vi "8-Tap 8-bit Camera with Serial Server(FPGA).vi"() -> ()   [LabVIEW 2013]
doc: "This is the FPGA VI for the 10-Tap 8-Bit Camera with DRAM example. This example demonstrates how to acquire images from a 10-tap, 8-bit, extended configuration, Camera Link camera and transfer the images to the host. This example supports area scan and line scan cameras for both continuous and finite acquisitions.\n\nThis example also demonstrates the use of DRAM as a frame buffer for very high speed acquisitions. Data packing and flow-control are also employed to maximize use of the available DRAM and FIFOs in terms of both memory space and performance.\n\nAdditionally, the example demonstrates the serial server, which allows third-party camera configuration utilities to communicate with the camera using the Camera Link serial interface while this VI is running."
uses:
  Common/CL Signal Mapping.ctl
  Common/CL Configuration.ctl
  FPGA/Sector/Accumulate/Sector Parameter Cluster.ctl
  <vilib>/Platform/TimedLoop/XDataNode/timing_clust.ctl
  <vilib>/Platform/TimedLoop/XDataNode/nitl_modes.ctl
  <vilib>/Platform/TimedLoop/XDataNode/wakeup.ctl
  <vilib>/rvi/Emulation/niFpgaSctlEmulationGetInTimedLoop.vi
  <vilib>/rvi/Emulation/niFpgaEmulationReportErrorSimple.vi
  <vilib>/rvi/eio/common/nirviEmuTemplateMethod_errors.vi
  <vilib>/rvi/Emulation/niFpgaGetClockAttributes.vi
  <vilib>/rvi/Emulation/niFpgaCriticalErrorInLSC.vi
  Common/CL Data to Pixels/8 Tap 8-Bit.vi
  FPGA/Globals/Accumulated Sector Intensity.vi
  <vilib>/rvi/FIFO/Fifo_Resource/nirvififoEmulationWriteFpgaImpl.vi
  <vilib>/rvi/DataTransferAndStorage/Container/Common/niFpgaContainerGetUniqueNameForEmu.vi
  <vilib>/rvi/interface/RandomDataEmulation/nirviRandomDataFPGAFIFO.vi
  <vilib>/rvi/interface/RandomDataEmulation/niFpgaRandomDataHandleErrors.vi
  <vilib>/rvi/FIFO/Fifo_Resource/nirvififoEmulationGetNumberOfElementsToReadFpgaImpl.vi
  <vilib>/rvi/FIFO/Fifo_Resource/nirvififoEmulationGetNumberOfElementsToWriteFpgaImpl.vi
  <vilib>/rvi/FIFO/Fifo_Resource/nirvififoEmulationReadFpgaImpl.vi
  FPGA/Globals/Sector Parameter Global.vi
  <vilib>/rvi/Emulation/niFpgaProcessEmulError.vi
  FPGA/Globals/Pixel Location Global.vi
  <vilib>/Platform/TimedLoop/XDataNode/XDataNode.xnode
  <vilib>/eio/EIONode/EIONode.xnode
  <vilib>/rvi/DataTransferAndStorage/Container/XNode/niFpgaContainer.xnode
  <vilib>/rvi/FIFO/Fifo_Resource/nirvififoEmulationWrite.vi
  <vilib>/rvi/interface/RandomDataEmulation/nirviRandomDataFpgaReadWriteTemplate.vi
  <vilib>/rvi/FIFO/Fifo_Resource/nirvififoEmulationGetNumberOfElementsToRead.vi
  <vilib>/rvi/FIFO/Fifo_Resource/nirvififoEmulationGetNumberOfElementsToWrite.vi
  <vilib>/rvi/FIFO/Fifo_Resource/nirvififoEmulationRead.vi
  <vilib>/Platform/TimedLoop/XDataNode/XDNodeRunTimeDep.lvlib
panel:
  out "Analysis Ticks":u32
  out "Right Sector Edge":u16
  out "Left Sector Edge":u16
  in  "# of Frames to Average":u8
  in  "Sector Parameters Left":T1={"Start Angle"=0.65740966796875, "End Angle"=0.99468994140625, "Inner Radius"=309, "Outter Radius"=405, "Hinge X"=464, "Hinge Y"=534, "NumWingSectors"=8}
  in  "Sector Parameters Right":T1={"Start Angle"=0.0, "End Angle"=0.4708251953125, "Inner Radius"=309, "Outter Radius"=405, "Hinge X"=685, "Hinge Y"=527, "NumWingSectors"=8}
  in  "Sector Threshold":u8
  in  "[Average BG Intensity]":u8[](array[numeric])=[0, 0, 0, 0, 0, 0, 0, 0, 0, 0, 0, 0, 0, 0, 0, 0, 0, 0, 0, 0, 0, 0, 0, 0, 0, 0, 0, 0, 0, 0, 0, 0]
  in  "X Resolution":u16=1000
  in  "Y Resolution":u16=1000
  in  "Left Start Angle Duty Cycle":fxp<+,8,0>
  in  "Left End Angle Duty Cycle":fxp<+,8,0>
  in  "Right Start Angle Duty Cycle":fxp<+,8,0>
  in  "Right End Angle Duty Cycle":fxp<+,8,0>
  out "Number of Elements to Write Host DMA":u32
  out "Number of Elements to Read Cam Data":u32
  in  "CL Config.Configuration":T2=enum."Full"
  in  "CL Config.Signal Mapping":T3
  in  "CL Config.Line Scan":bool
  in  "CL Config.DVAL Active High":bool=TRUE
  in  "CL Config.LVAL Active High":bool=TRUE
  in  "CL Config.FVAL Active High":bool=TRUE
  in  "CL Config.Spare Active High":bool=TRUE
  in  "Acq Control.Line Scan Height":u32
  in  "Acq Control.Frames To Acq":u32
  in  "Acq Control.Acquire":bool
  in  "Acq Control.Cancel Acq":bool
  in  "Acq Control.Ignore DVAL":bool
  in  "Acq Control.Initialize":bool
  out "Acq Status.Acq In Progress":bool
  out "Acq Status.Clocks Per Line":u32
  out "Acq Status.Frames Acq'd":u32
  out "Acq Status.Lines Per Frame":u32
  out "Acq Status.DMA Write Timeout":bool
  out "Acq Status.Initialized":bool
  in  "UART.Baud Rate":u8
  in  "UART.Transmit":bool
  in  "UART.Tx Data":u8[](array[numeric])=[0, 0, 0, 0, 0, 0, 0, 0, 0, 0] format="%02x"
  in  "UART.Set Baud Rate":bool
  in  "UART.Byte Mode":bool=TRUE
  out "UART.Rx Ready":bool
  out "UART.Break Indicator":bool
  out "UART.Framing Error":bool
  out "UART.Overrun Error":bool
  out "UART.Tx Ready":bool
  out "UART.Rx Data":u8 format="%02x"
  in  "UART.Receive":bool
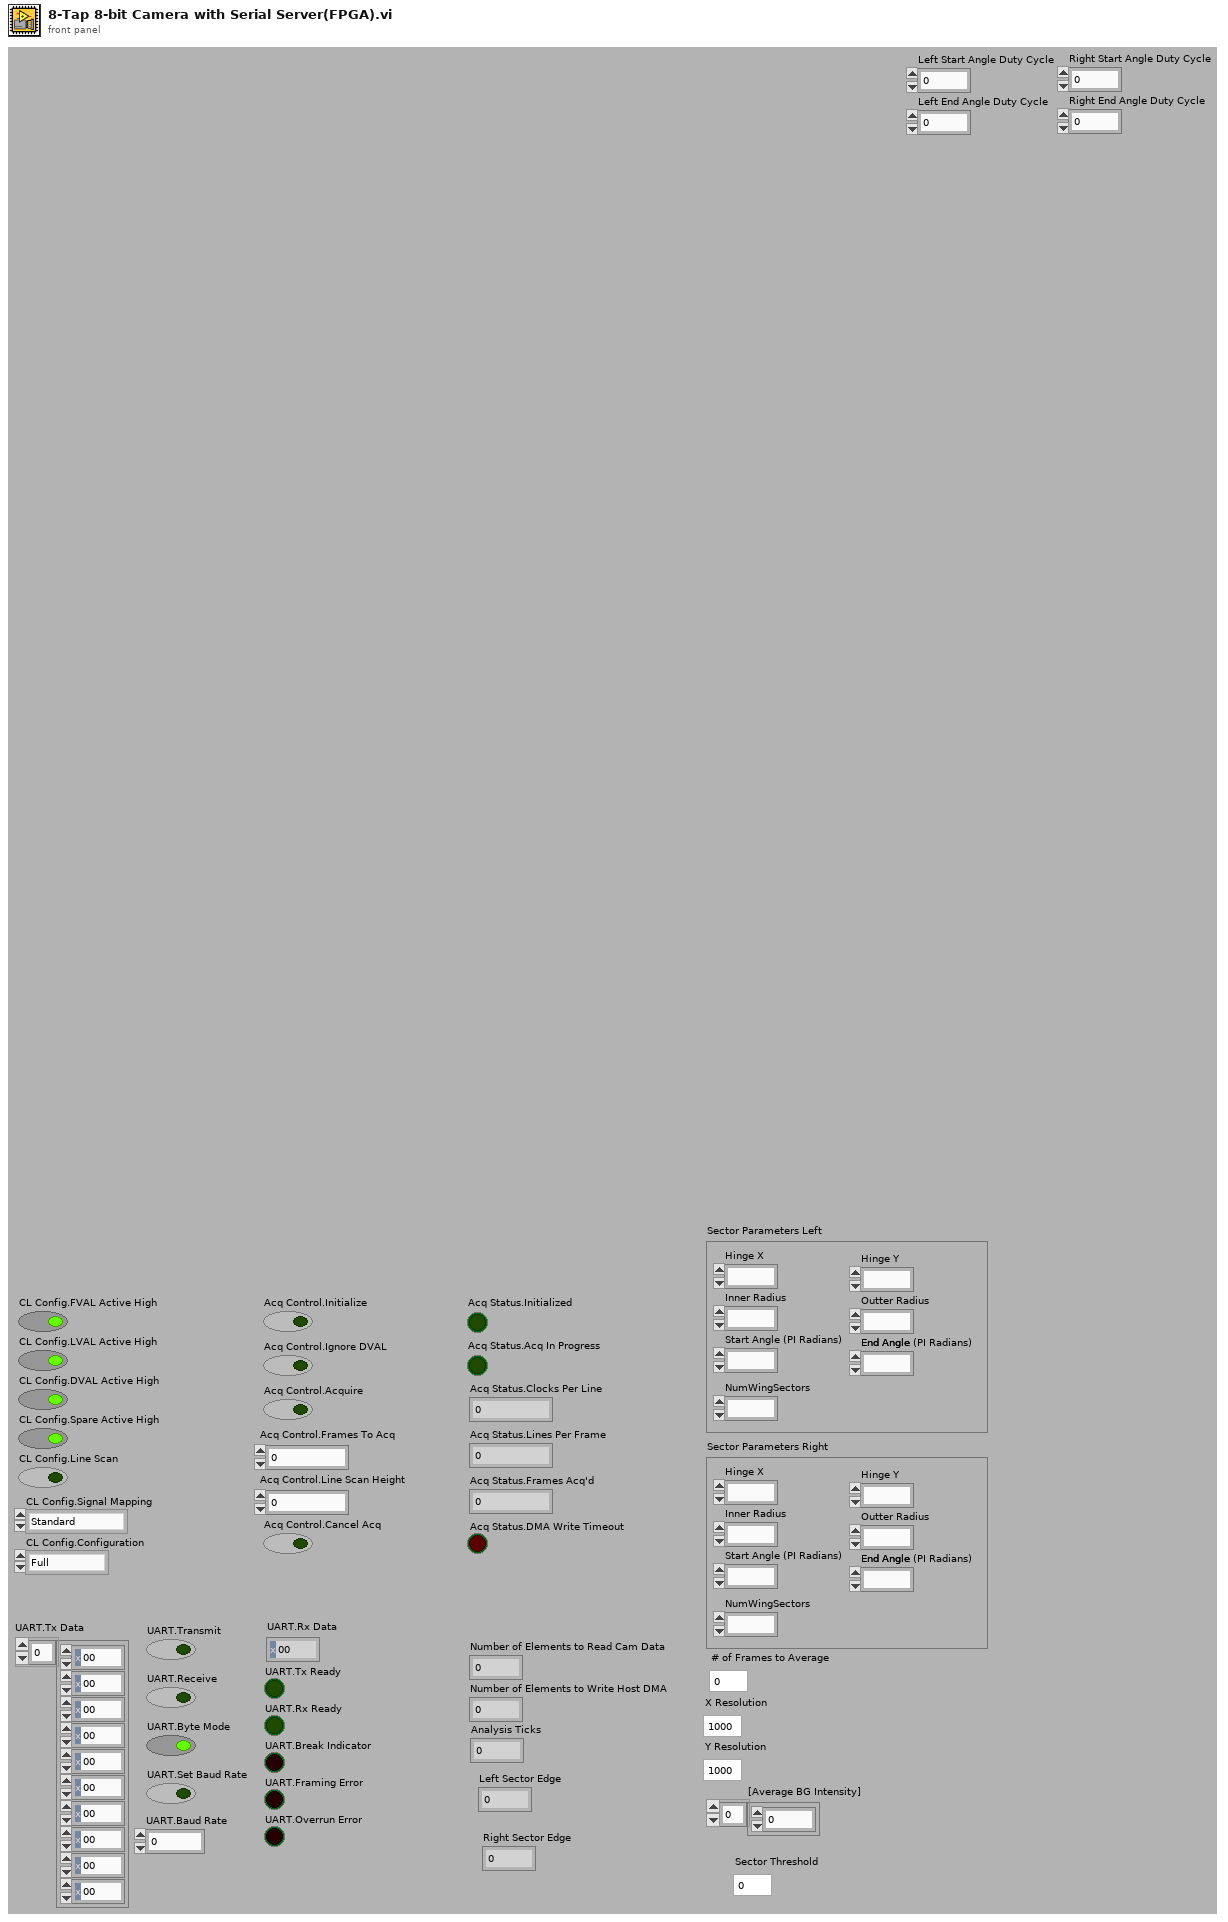
[diagram p1: front panel]
types:
  T1 = typedef "Sector Parameter Cluster.ctl" = cluster{"Start Angle":fxp<+/-,17,2>, "End Angle":fxp<+/-,17,2>, "Inner Radius":u16, "Outter Radius":u16, "Hinge X":u16, "Hinge Y":u16, "NumWingSectors":u8}
  T2 = typedef "CL Configuration.ctl" = enum8{"Base", "Medium", "Full"}
  T3 = typedef "CL Signal Mapping.ctl" = enum8{"Standard", "Basler 10-tap", "Vosskühler 10-tap"}
  T4 = typedef "XDNodeRunTimeDep.lvlib/timing_clust.ctl" = cluster{"Expected End [f-1]":u64, "Actual End [f-1]":u64, "Finished Late? [f-1]":bool, "Expected End [i-1]":u64, "Actual End [i-1]":u64, "Finished Late? [i-1]":bool, "Expected Start [i]":u64, "Actual Start [i]":u64, "Expected Start [f]":u64, "Actual Start [f]":u64, "Source Name":string, "Structure Name":string, "Period":i64, "Deadline":i64, "Offset":i64, "Start":i64, "Priority":i32, "Timeout":i32, "Mode":T5, "Wakeup Reason":T6, "Error":errorcluster, "Source Type":string, "Secondary Source Type":string, "Global End Time":u64, "Global Start Time":u64, "Frame Duration":u64, "Iteration Duration":u64, "Assigned CPU":i32, "I/O Scan Engine Mode":u32}
  T5 = typedef "XDNodeRunTimeDep.lvlib/nitl_modes.ctl" = enum32{"No Change", "Process missed periods, maintain original phase", "Discard missed periods, maintain original phase", "Process missed periods, ignore original phase", "Discard missed periods, ignore original phase"}
  T6 = typedef "XDNodeRunTimeDep.lvlib/wakeup.ctl" = enum32{"Normal", "Aborted", "Asynchronous wakeup", "Timing source error", "Timed loop error", "Timeout"}
  T7 = cluster{"Enables Valid":bool, "Frame Valid":bool, "Line Valid":bool, "Data Valid":bool}
  T8 = cluster{"Pixel 0":u8, "Pixel 1":u8, "Pixel 2":u8, "Pixel 3":u8, "Pixel 4":u8, "Pixel 5":u8, "Pixel 6":u8, "Pixel 7":u8}
  T9 = cluster{"Tx Data":u8[], "Transmit":bool, "Receive":bool, "Byte Mode":bool, "Set Baud Rate":bool, "Baud Rate":u8}
  T10 = cluster{"Rx Data":u8, "Turn Off Transmit":bool, "Turn Off Receive":bool, "Turn Off Set Baud Rate":bool, "Tx Ready":bool, "Rx Ready":bool, "Break Indicator":bool, "Framing Error":bool, "Overrun Error":bool}
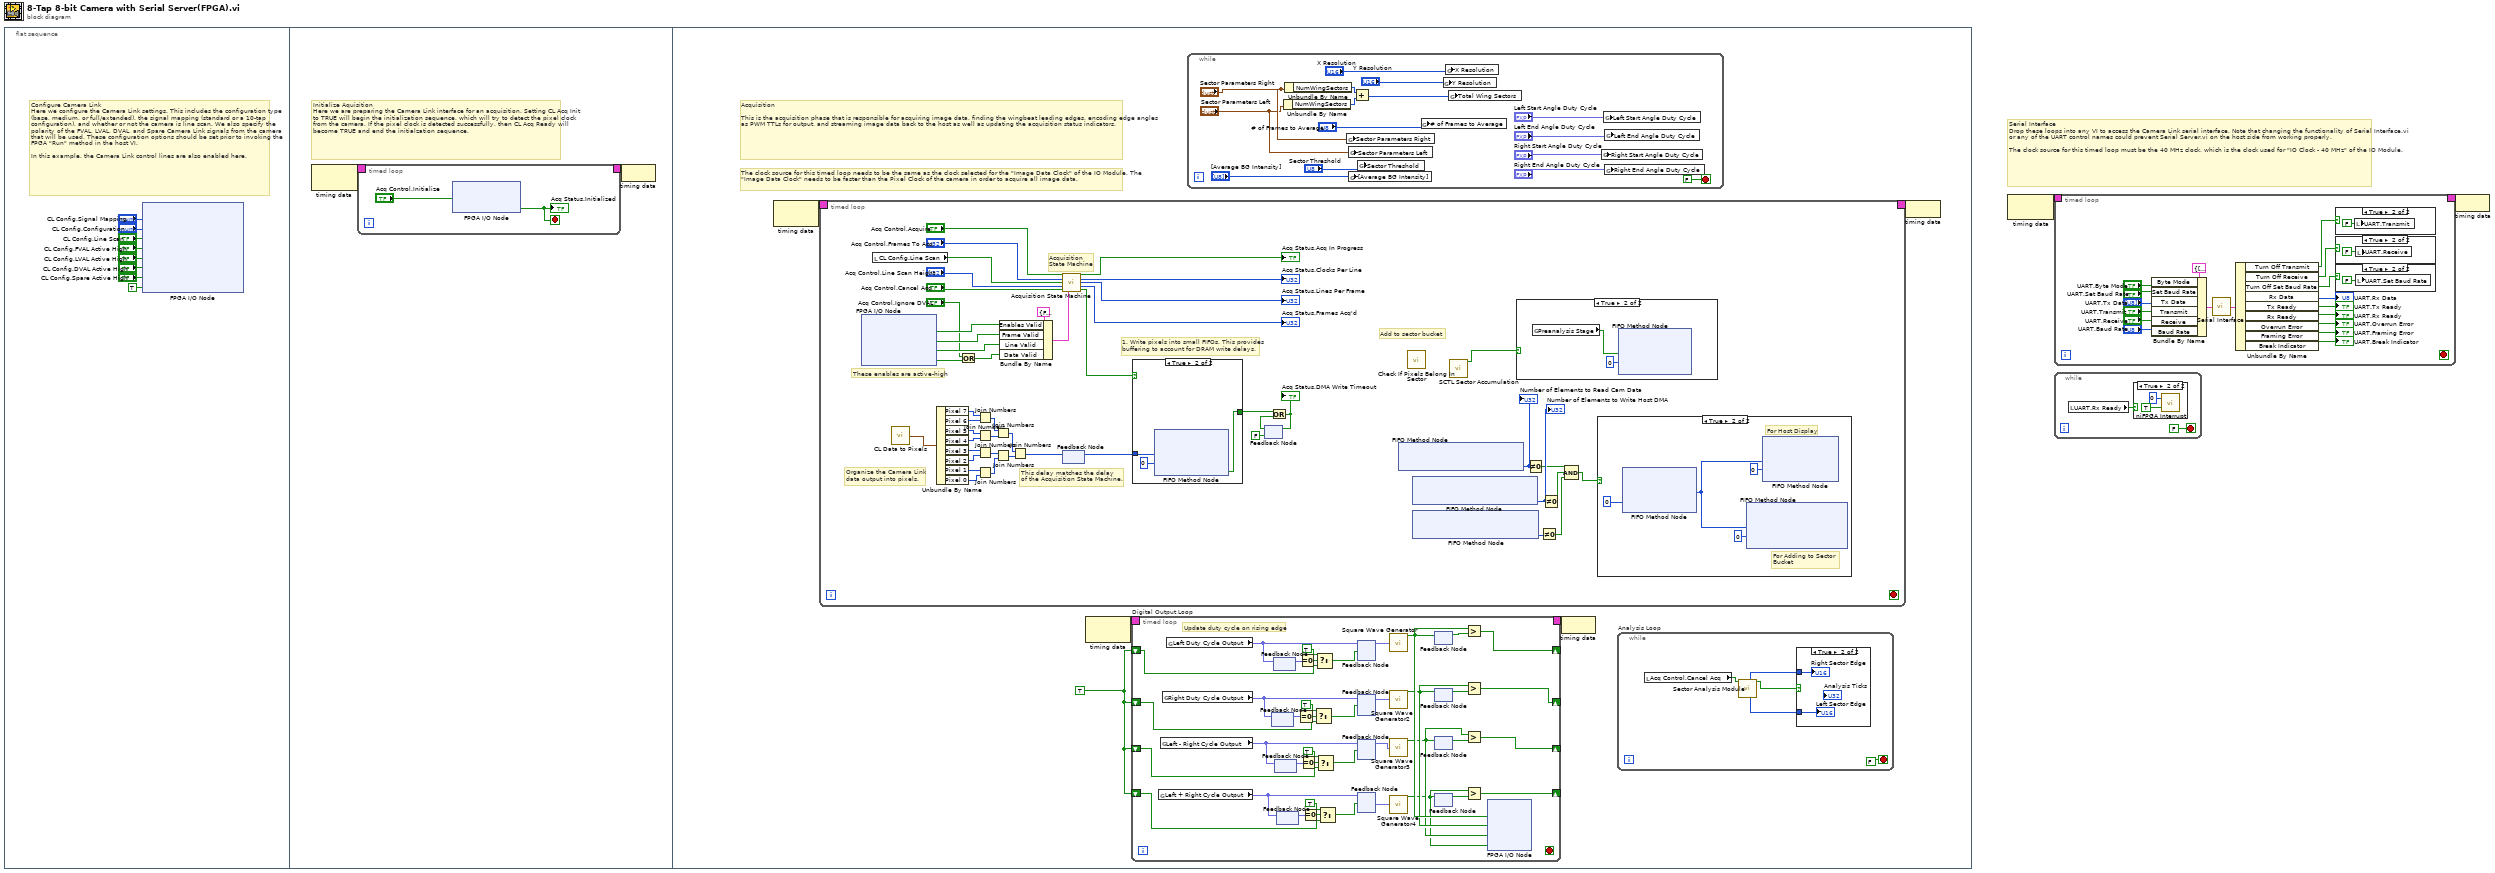
[diagram p0: block diagram]
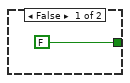
[diagram p9: hidden frame]
diagram:
  # "Serial Interface\nDrop these loops into any VI to access the Camera Link serial interface. Note that changing the functionality of Serial Interface.vi or any of the UART control names could prevent Serial Server.vi on the host side from working properly.\n\nThe clock source for this timed loop must be the 40 MHz clock, which is the clock used for \"IO Clock - 40 MHz\" of the IO Module."
  n1 = flat-sequence {
    frame #0 {
      # "Configure Camera Link\nHere we configure the Camera Link settings. This includes the configuration type (base, medium, or full/extended), the signal mapping (standard or a 10-tap configuration), and whether or not the camera is line scan. We also specify the polarity of the FVAL, LVAL, DVAL, and Spare Camera Link signals from the camera that will be used. These configuration options should be set prior to invoking the FPGA \"Run\" method in the host VI.\n\nIn this example, the Camera Link control lines are also enabled here."
      n2 = xnode "FPGA I/O Node"("CL Set Signal Mapping"="CL Config.Signal Mapping", "CL Set Configuration"="CL Config.Configuration", "CL Set Line Scan"="CL Config.Line Scan", "CL Set FVAL Active High"="CL Config.FVAL Active High", "CL Set LVAL Active High"="CL Config.LVAL Active High", "CL Set DVAL Active High"="CL Config.DVAL Active High", "CL Set Spare Active High"="CL Config.Spare Active High", "CL Control Enable"=TRUE ("IO Module\\CL Control Enable")) -> ()  [unwired: 8 in, 8 out]
    }
    frame #1 {
      # "Initialize Aquisition\nHere we are preparing the Camera Link interface for an acquisition. Setting CL Acq Init to TRUE will begin the initialization sequence, which will try to detect the pixel clock from the camera. If the pixel clock is detected successfully, then CL Acq Ready will become TRUE and end the initialzation sequence."
      n3 = node-c288() -> (w12:T4)  [unwired: 1 out]
      n4 = timed-loop {
        timing: w12 -> [_]
        timing-out: [_] -> w11
        stop <- w13 stop-if-true
        n5 = xnode "FPGA I/O Node"("CL Acq Init"="Acq Control.Initialize") -> ("CL Acq Ready"=w13:bool)  [unwired: 2 in, 2 out]
        "Acq Status.Initialized" <- w13
      }
      n6 = node-c288(w11) -> ()
    }
    frame #2 {
      w19 = TRUE
      # "The clock source for this timed loop needs to be the same as the clock selected for the \"Image Data Clock\" of the IO Module. The \"Image Data Clock\" needs to be faster than the Pixel Clock of the camera in order to acquire all image data."
      # "Acquisition\n\nThis is the acquisition phase that is responsible for acquiring image data, finding the wingbeat leading edges, encoding edge angles as PWM TTLs for output, and streaming image data back to the host as well as updating the acquisition status indicators."
      n7 = node-c288() -> (w23:T4)  [unwired: 1 in]
      n8 = timed-loop {
        timing: w23 -> [_]
        timing-out: [_] -> w22
        stop <- _ stop-if-true
        # "Add to sector bucket"
        # "1. Write pixels into small FIFOs. This provides\nbuffering to account for DRAM write delays."
        # "Organize the Camera Link\ndata output into pixels."
        # "These enables are active-high"
        # "This delay matches the delay\nof the Acquisition State Machine."
        # "Acquisition\nState Machine"
        n9 = xnode "FPGA I/O Node"() -> ("CL Output Valid"=w122:bool, "CL Frame Valid"=w121:bool, "CL Line Valid"=w120:bool, "CL Data Valid"=w117:bool)  [unwired: 4 in, 4 out]
        n10 = local read "CL Config.Line Scan"() -> (w114:bool)
        n11 = call-poly "CL Data to Pixels.vi"() -> ("Pixels"=w136:T8)  [unwired: 1 in]
        n12 = Unbundle By Name(w136) -> ("Pixel 7"=w112:u8, "Pixel 6"=w111:u8, "Pixel 5"=w110:u8, "Pixel 4"=w109:u8, "Pixel 3"=w108:u8, "Pixel 2"=w107:u8, "Pixel 1"=w106:u8, "Pixel 0"=w105:u8)
        n13 = Or(x="Acq Control.Ignore DVAL", y=w117) -> (x .or. y?=w116:bool)
        n14 = Join Numbers(hi=w112, lo=w111) -> ((hi.lo)=w103:u16)
        n15 = Join Numbers(hi=w110, lo=w109) -> ((hi.lo)=w102:u16)
        n16 = Join Numbers(hi=w108, lo=w107) -> ((hi.lo)=w101:u16)
        n17 = Join Numbers(hi=w106, lo=w105) -> ((hi.lo)=w104:u16)
        n18 = Join Numbers(hi=w103, lo=w102) -> ((hi.lo)=w100:u32)
        n19 = Join Numbers(hi=w101, lo=w104) -> ((hi.lo)=w99:u32)
        n20 = Bundle By Name(cluster=T7 {"Enables Valid"=FALSE, "Frame Valid"=FALSE, "Line Valid"=FALSE, "Data Valid"=FALSE} ("Enables"), "Enables Valid"=w122, "Frame Valid"=w121, "Line Valid"=w120, "Data Valid"=w116) -> (w119:T7)
        n21 = Join Numbers(hi=w100, lo=w99) -> ((hi.lo)=w98:u64)
        n22 = call "Acquisition State Machine.vi"("Acquire"="Acq Control.Acquire", "Frames to Acquire"="Acq Control.Frames To Acq", "Line Scan"=w114, "Line Scan Height"="Acq Control.Line Scan Height", "Cancel Acq"="Acq Control.Cancel Acq", "Enables"=w119) -> ("Acq In Progress"=→"Acq Status.Acq In Progress":bool, "Num Clocks Per Line"=→"Acq Status.Clocks Per Line":u32, "Num Lines Per Frame"=→"Acq Status.Lines Per Frame":u32, "Num Frames Acq'd"=→"Acq Status.Frames Acq'd":u32, "Capture Cycle"=w134:bool)  [unwired: 4 in, 1 out]
        n23 = feedback-in #1(w98) -> ()
        n24 = feedback #1() -> (w135:u64)  [unwired: 1 in]
        n25 = case shown="True" w134 {
          tunnel: [FALSE ("Timed Out?") w145] -> w132
          tunnel: w135 -> [_ w146]
          frame False {
          }
          frame True {
            n26 = xnode ("FIFO Method Node")("Element"=w146, "Timeout"=0) -> ("Timed Out?"=w145:bool)  [unwired: 1 in, 1 out]
          }
        }
        n27 = feedback #2(FALSE) -> (w131:bool)
        n28 = Or(x=w132, y=w131) -> (x .or. y?=w130:bool)
        "Acq Status.DMA Write Timeout" <- w130
        n29 = feedback-in #2(w130) -> ()
        n30 = xnode ("FIFO Method Node")() -> ("Number of Elements to Read"=w96:u32)  [unwired: 1 in, 1 out]
        "Number of Elements to Read Cam Data" <- w96
        n31 = call "Check If Pixels Belong In Sector.vi"() -> ()  [unwired: 11 in, 1 out]
        n32 = xnode ("FIFO Method Node")() -> ("Number of Elements to Write"=w94:u32)  [unwired: 1 in, 1 out]
        "Number of Elements to Write Host DMA" <- w94
        n33 = xnode ("FIFO Method Node")() -> ("Number of Elements to Write"=w93:u32)  [unwired: 1 in, 1 out]
        n34 = call "SCTL Sector Accumulation.vi"() -> ("New Data?"=w97:bool)  [unwired: 10 in, 1 out]
        n35 = case shown="True" w97 {
          frame False {
          }
          frame True {
            n36 = global read "Accumulated Sector Intensity.vi" "Preanalysis Stage"() -> (w141:bool)
            n37 = xnode ("FIFO Method Node")("Element"=w141, "Timeout"=0) -> ()  [unwired: 1 in, 2 out]
          }
        }
        n38 = Not Equal To 0?(x=w96) -> (x != 0?=w91:bool)
        n39 = Not Equal To 0?(x=w93) -> (x != 0?=w92:bool)
        n40 = Not Equal To 0?(x=w94) -> (x != 0?=w95:bool)
        n41 = Compound Arithmetic op=AND(w91, w95, w92) -> (w90:bool)
        n42 = case shown="True" w90 {
          frame False {
          }
          frame True {
            # "For Adding to Sector \nBucket"
            # "For Host Display"
            n43 = xnode ("FIFO Method Node")("Timeout"=0) -> ("Element"=w137:u64)  [unwired: 1 in, 2 out]
            n44 = xnode ("FIFO Method Node")("Element"=w137, "Timeout"=0) -> ()  [unwired: 1 in, 2 out]
            n45 = xnode ("FIFO Method Node")("Element"=w137, "Timeout"=0) -> ()  [unwired: 1 in, 2 out]
          }
        }
      }
      n46 = node-c288() -> (w21:T4)  [unwired: 1 in]
      n47 = timed-loop "Digital Output Loop" {
        timing: w21 -> [_]
        timing-out: [_] -> w20
        shift-right: [w79] -> _
        shift-left: w19 -> [w64]
        shift-right: [w78] -> _
        shift-left: w19 -> [w50]
        shift-right: [w77] -> _
        shift-left: w19 -> [w48]
        shift-right: [w71] -> _
        shift-left: w19 -> [w46]
        stop <- _ stop-if-true
        # "Update duty cycle on rising edge"
        n48 = global read "Sector Parameter Global.vi" "Left + Right Cycle Output"() -> (w52:fxp<+,8,0>)
        n49 = global read "Sector Parameter Global.vi" "Left - Right Cycle Output"() -> (w53:fxp<+,8,0>)
        n50 = global read "Sector Parameter Global.vi" "Right Duty Cycle Output"() -> (w54:fxp<+/-,9,1>)
        n51 = global read "Sector Parameter Global.vi" "Left Duty Cycle Output"() -> (w67:fxp<+/-,9,1>)
        n52 = feedback #3() -> (w61:fxp<+/-,9,1>)  [unwired: 1 in]
        n53 = feedback-in #3(w54) -> ()
        n54 = feedback #4() -> (w66:fxp<+/-,9,1>)  [unwired: 1 in]
        n55 = feedback-in #4(w67) -> ()
        n56 = feedback #5() -> (w58:fxp<+,8,0>)  [unwired: 1 in]
        n57 = feedback-in #5(w53) -> ()
        n58 = feedback #6() -> (w55:fxp<+,8,0>)  [unwired: 1 in]
        n59 = feedback-in #6(w52) -> ()
        n60 = Equal To 0?(x=w61) -> (x = 0?=w62:bool)
        n61 = Equal To 0?(x=w66) -> (x = 0?=w68:bool)
        n62 = Equal To 0?(x=w58) -> (x = 0?=w59:bool)
        n63 = Equal To 0?(x=w55) -> (x = 0?=w56:bool)
        n64 = Select(t=TRUE, s=w62, f=w50) -> (s? t:f=w51:bool)
        n65 = Select(t=TRUE, s=w68, f=w64) -> (s? t:f=w65:bool)
        n66 = Select(t=TRUE, s=w59, f=w48) -> (s? t:f=w49:bool)
        n67 = Select(t=TRUE, s=w56, f=w46) -> (s? t:f=w47:bool)
        n68 = feedback-in #7(w67, w65) -> ()
        n69 = feedback #7() -> (w85:fxp<+/-,9,1>)  [unwired: 1 in]
        n70 = feedback #8() -> (w84:fxp<+/-,9,1>)  [unwired: 1 in]
        n71 = feedback-in #8(w54, w51) -> ()
        n72 = feedback #9() -> (w83:fxp<+,8,0>)  [unwired: 1 in]
        n73 = feedback-in #9(w53, w49) -> ()
        n74 = feedback #10() -> (w73:fxp<+,8,0>)  [unwired: 1 in]
        n75 = feedback-in #10(w52, w47) -> ()
        n76 = call "Square Wave Generator"("duty cycle (periods)"=w85) -> ("square wave out"=w76:bool)  [unwired: 14 in]
        n77 = call "Square Wave Generator2"("duty cycle (periods)"=w84) -> ("square wave out"=w75:bool)  [unwired: 14 in]
        n78 = call "Square Wave Generator3"("duty cycle (periods)"=w83) -> ("square wave out"=w74:bool)  [unwired: 14 in]
        n79 = call "Square Wave Generator4"("duty cycle (periods)"=w73) -> ("square wave out"=w70:bool)  [unwired: 14 in]
        n80 = feedback-in #11(w76) -> ()
        n81 = feedback #11() -> (w82:bool)  [unwired: 1 in]
        n82 = feedback #12() -> (w81:bool)  [unwired: 1 in]
        n83 = feedback-in #12(w75) -> ()
        n84 = feedback #13() -> (w80:bool)  [unwired: 1 in]
        n85 = feedback-in #13(w74) -> ()
        n86 = feedback #14() -> (w72:bool)  [unwired: 1 in]
        n87 = feedback-in #14(w70) -> ()
        n88 = Greater?(x=w76, y=w82) -> (0:w79:bool)
        n89 = Greater?(x=w75, y=w81) -> (0:w78:bool)
        n90 = Greater?(x=w74, y=w80) -> (0:w77:bool)
        n91 = Greater?(x=w70, y=w72) -> (0:w71:bool)
        n92 = xnode "FPGA I/O Node"("TTL 1"=w76, "TTL 2"=w75, "TTL 3"=w74, "TTL 4"=w70) -> ()  [unwired: 4 in, 4 out]
      }
      n93 = while {
        stop <- FALSE stop-if-true
        n94 = Unbundle By Name("Sector Parameters Left") -> ("NumWingSectors"=w43:u8)
        n95 = Unbundle By Name("Sector Parameters Right") -> ("NumWingSectors"=w44:u8)
        n96 = global write "Sector Parameter Global.vi" "Sector Parameters Right"("Sector Parameters Right") -> ()
        n97 = global write "Sector Parameter Global.vi" "Sector Parameters Left"("Sector Parameters Left") -> ()
        n98 = global write "Sector Parameter Global.vi" "[Average BG Intensity]"("[Average BG Intensity]") -> ()
        n99 = Add(x=w44, y=w43) -> (x+y=w42:u8)
        n100 = global write "Sector Parameter Global.vi" "Sector Threshold"("Sector Threshold") -> ()
        n101 = global write "Pixel Location Global.vi" "# of Frames to Average"("# of Frames to Average") -> ()
        n102 = global write "Pixel Location Global.vi" "Y Resolution"("Y Resolution") -> ()
        n103 = global write "Pixel Location Global.vi" "X Resolution"("X Resolution") -> ()
        n104 = global write "Accumulated Sector Intensity.vi" "Total Wing Sectors"(w42) -> ()
        n105 = global write "Sector Parameter Global.vi" "Right Start Angle Duty Cycle"("Right Start Angle Duty Cycle") -> ()
        n106 = global write "Sector Parameter Global.vi" "Left Start Angle Duty Cycle"("Left Start Angle Duty Cycle") -> ()
        n107 = global write "Sector Parameter Global.vi" "Left End Angle Duty Cycle"("Left End Angle Duty Cycle") -> ()
        n108 = global write "Sector Parameter Global.vi" "Right End Angle Duty Cycle"("Right End Angle Duty Cycle") -> ()
      }
      n109 = node-c288(w20) -> ()
      n110 = while "Analysis Loop" {
        stop <- FALSE stop-if-true
        n111 = local read "Acq Control.Cancel Acq"() -> (w27:bool)
        n112 = call "Sector Analysis Module.vi"("Canceled?"=w27) -> ("Data"=w24:bool, "Left Sector Edge"=w25:u16, "Right Sector Edge"=w26:u16)  [unwired: 7 in, 1 out]
        n113 = case shown="True" w24 {
          tunnel: w26 -> [_ w30]
          tunnel: w25 -> [_ w29]
          frame False {
          }
          frame True {
            "Right Sector Edge" <- w30
            "Left Sector Edge" <- w29
          }
        }
      }
      n114 = node-c288(w22) -> ()
    }
  }
  n115 = node-c288() -> (w2:T4)  [unwired: 1 out]
  n116 = timed-loop {
    timing: w2 -> [_]
    timing-out: [_] -> w1
    stop <- _ stop-if-true
    n117 = Bundle By Name(cluster=T9 {"Tx Data"=[0, 0, 0, 0, 0, 0, 0, 0, 0, 0], "Transmit"=FALSE, "Receive"=FALSE, "Byte Mode"=TRUE, "Set Baud Rate"=FALSE, "Baud Rate"=0} ("UART Inputs"), "Byte Mode"="UART.Byte Mode", "Set Baud Rate"="UART.Set Baud Rate", "Tx Data"="UART.Tx Data", "Transmit"="UART.Transmit", "Receive"="UART.Receive", "Baud Rate"="UART.Baud Rate") -> (w151:T9)
    n118 = call "Serial Interface.vi"("UART Inputs"=w151) -> ("UART Outputs"=w163:T10)
    n119 = Unbundle By Name(w163) -> ("Turn Off Transmit"=w156:bool, "Turn Off Receive"=w157:bool, "Turn Off Set Baud Rate"=w153:bool, "Rx Data"=→"UART.Rx Data":u8, "Tx Ready"=→"UART.Tx Ready":bool, "Rx Ready"=→"UART.Rx Ready":bool, "Overrun Error"=→"UART.Overrun Error":bool, "Framing Error"=→"UART.Framing Error":bool, "Break Indicator"=→"UART.Break Indicator":bool)
    n120 = case shown="True" w156 {
      frame False {
      }
      frame True {
        n121 = local write "UART.Transmit"(FALSE ("UART.Transmit")) -> ()
      }
    }
    n122 = case shown="True" w157 {
      frame False {
      }
      frame True {
        n123 = local write "UART.Receive"(FALSE ("UART.Receive")) -> ()
      }
    }
    n124 = case shown="True" w153 {
      frame False {
      }
      frame True {
        n125 = local write "UART.Set Baud Rate"(FALSE ("UART.Receive")) -> ()
      }
    }
  }
  n126 = while {
    stop <- FALSE stop-if-true
    n127 = local read "UART.Rx Ready"() -> (w175:bool)
    n128 = case shown="True" w175 {
      frame False {
      }
      frame True {
        n129 = call <vilib>:"niFPGA Interrupt.vi"("Wait Until Cleared (F)"=TRUE ("Wait Until Cleared"), "IRQ Number (0)"=u8 0 ("IRQ Number")) -> ()  [unwired: 1 in]
      }
    }
  }
  n130 = node-c288(w1) -> ()
